vi "Get Properties.vi"(8 "error in":errorcluster) -> (0 "error out":errorcluster, 3 "logger properties":T2(array[cluster]))   [LabVIEW 2018, in "GLog.lvlib"]
doc: "Get the Name, Minimum Log Level, and Enabled state of all currently registered loggers in the Registry."
uses:
  GLog.lvlib
  logger_class/Log Levels.ctl
  registry/Registry.lvlib
  logger_class/Logger.lvclass
panel:
  # "Connector Pane"
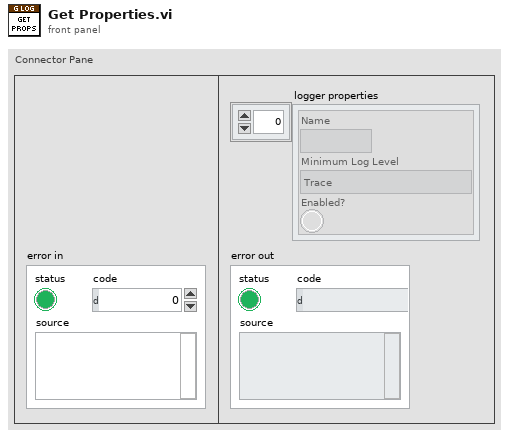
[diagram p1: front panel]
types:
  T1 = typedef "GLog.lvlib/Logger.lvclass/Log Levels.ctl" = enum16{"Trace", "Debug", "Info", "Warning", "Error", "Critical"}
  T2 = cluster{"Name":string, "Minimum Log Level":T1, "Enabled?":bool}[]
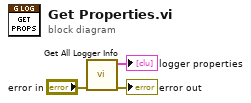
[diagram p0: block diagram]
diagram:
  n1 = call "Get All Logger Info.vi"("error in"="error in") -> ("error out"=→"error out":errorcluster, "logger info"=→"logger properties":T2)  [unwired: 9 in]
